vi "Auto_Drive_Test.vi"(8 "Timer?":bool, 9 "Duration":u32=3500, 10 "distance":dbl=88.0 format="%#_13g", 11 "Drive Effort":dbl=1000.0) -> ()   [LabVIEW 2016]
uses:
  <vilib>/Rock Robotics/WPI/SafetyOutput/WPI_SafetyOutputConfigMenu.ctl
panel:
  in  "Max Error":dbl=100.0 format="%#_13g"
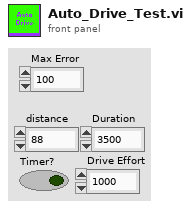
[diagram p1: front panel]
types:
  T1 = typedef "WPI_SafetyOutputConfigMenu.ctl" = enum16{"Enable", "Disable"}
  T2 = typedef "WPI_MotorControlDeviceRef.ctl" = cluster{"DeviceStatus":errorcluster, "Type":T3, "PWM":cluster{"PWM Channel":T4, "DeadBand":T5}, "CAN":cluster{"Device Number":u8, "SetOutput VI Ref":variant, "GetOutput VI Ref":variant, "Enable VI Ref":variant, "Disable VI Ref":variant, "Data":variant}, "Invert":bool}
  T3 = typedef "WPI_MotorControlType.ctl" = enum16{"PWM", "CAN"}
  T4 = typedef "FPGA_DIOPWMChannel.ctl" = enum8{"PWM 0", "PWM 1", "PWM 2", "PWM 3", "PWM 4", "PWM 5", "PWM 6", "PWM 7", "PWM 8", "PWM 9", "PWM MXP 0", "PWM MXP 1", "PWM MXP 2", "PWM MXP 3", "PWM MXP 4", "PWM MXP 5", "PWM MXP 6", "PWM MXP 7", "PWM MXP 8", "PWM MXP 9", "Invalid"}
  T5 = typedef "WPI_PWMDeadband.ctl" = cluster{"Name":string, "maxPositivePwm":i32, "minPositivePwm":i32, "centerPwm":i32, "maxNegativePwm":i32, "minNegativePwm":i32, "angularRange":u16}
  T6 = typedef "WPI_CANTalonSRX_GlobalStatus.ctl" = cluster{"Applied Throttle":dbl, "Module Enabled":bool, "CAN Error":errorcluster, "Closed Loop Error":dbl, "Forward Limit Switch Closed":bool, "Reverse Limit Switch Closed":bool, "Sensor Position":dbl, "Sensor Velocity":dbl, "Current":dbl, "Sticky Fault - Over Temp":bool, "Sticky Fault - Under Voltage":bool, "Sticky Fault - Forward Limit":bool, "Sticky Fault - Reverse Limit":bool, "Sticky Fault - Forward Soft Limit":bool, "Sticky Fault - Reverse Soft Limit":bool, "Brake is Enabled":bool, "Encoder Position":dbl, "Encoder Velocity":dbl, "Encoder Index Count":dbl, "Encoder A Pin State":bool, "Encoder B Pin State":bool, "Encoder Index Pin State":bool, "Analog In":dbl, "Analog In Velocity":dbl, "Temperature (C)":dbl, "Battery Voltage":dbl, "Control 5 Is Supported":bool, "Current Profile Slot Select":dbl, "Pos Div 8":bool, "Vel Div 4":bool, "Pulse Width Position":i32, "Pulse Width Velocity":i32, "Pulse Width Rise To Rise (us)":i32, "Pulse Width Rise To Fall (us)":i32, "Mot Prof Active Is Under Run":bool, "Mot Prof Active Has Under Run":bool, "Mot Prof Active Is Last":bool, "Mot Prof Active Velocity Only":bool, "Mot Prof Active Is Valid":bool, "Mot Prof Buffer Is Full":bool, "Mot Prof Active Profile Slot Select":i32, "Mot Prof NextID":i32, "Mot Prof Count":i32, "Mot Prof Active Velocity":dbl, "Mot Prof Active Position":dbl, "Mot Prof Output Enable":i32}
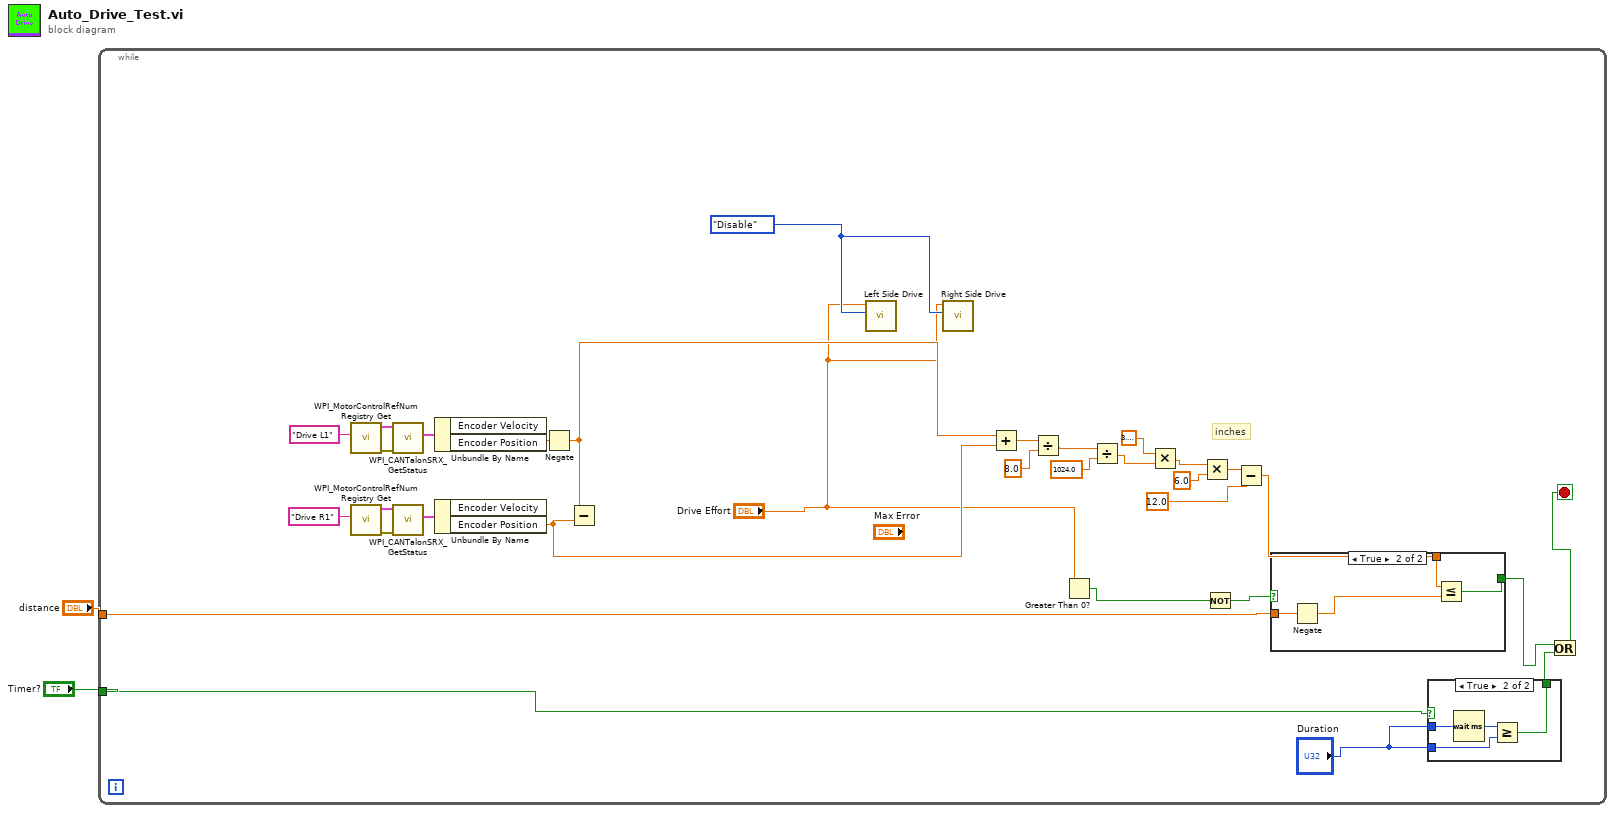
[diagram p0: block diagram]
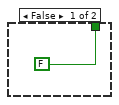
[diagram p2: hidden frame]
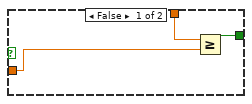
[diagram p3: hidden frame]
diagram:
  n1 = while {
    tunnel: "distance" -> [w18]
    tunnel: "Timer?" -> [w13]
    stop <- w10 stop-if-true
    w4 = WPI_SafetyOutputConfigMenu."Disable" ("mode")
    # "inches"
    n2 = call <vilib>:"WPI_MotorControlRefNum Registry Get.vi"("refnum name"="Drive L1") -> ("error out"=w29:errorcluster, "MotorControlDevRef"=w34:T2)  [unwired: 9 in]
    n3 = call <vilib>:"WPI_MotorControlRefNum Registry Get.vi"("refnum name"="Drive R1") -> ("error out"=w32:errorcluster, "MotorControlDevRef"=w33:T2)  [unwired: 9 in]
    n4 = call <vilib>:"WPI_CANTalonSRX_GetStatus.vi"("error in (no error)"=w29, "CAN Talon SRX Ref"=w34) -> ("Talon SRX Status"=w31:T6)  [unwired: 7 in, 2 out]
    n5 = call <vilib>:"WPI_CANTalonSRX_GetStatus.vi"("error in (no error)"=w32, "CAN Talon SRX Ref"=w33) -> ("Talon SRX Status"=w30:T6)  [unwired: 7 in, 2 out]
    n6 = Unbundle By Name(w31) -> ("Encoder Position"=w6:dbl)  [unwired: 1 out]
    n7 = Unbundle By Name(w30) -> ("Encoder Position"=w7:dbl)  [unwired: 1 out]
    n8 = Negate(x=w6) -> (-x=w5:dbl)
    n9 = Subtract(x=w5, y=w7) -> ()  [unwired: 1 out]
    n10 = call "Left Side Drive.vi"("mode"=w4, "Effort"="Drive Effort") -> ()  [unwired: 10 in]
    n11 = call "Right Side Drive.vi"("mode"=w4, "Effort"="Drive Effort") -> ()  [unwired: 10 in]
    n12 = Add(x=w5, y=w7) -> (x+y=w28:dbl)
    n13 = Divide(x=w28, y=8.0) -> (x/y=w26:dbl)
    n14 = Greater Than 0?(x="Drive Effort") -> (x > 0?=w14:bool)
    n15 = Divide(x=w26, y=1024.0) -> (x/y=w24:dbl)
    n16 = Multiply(x=3.141592653589793, y=w24) -> (x*y=w22:dbl)
    n17 = Multiply(x=w22, y=6.0) -> (x*y=w17:dbl)
    n18 = Not(x=w14) -> (.not. x?=w8:bool)
    n19 = Subtract(x=w17, y=12.0) -> (x-y=w15:dbl)
    n20 = case shown="True" w8 {
      tunnel: [w40 w46] -> w12
      tunnel: w18 -> [w41 w44]
      tunnel: w15 -> [w42 w43]
      frame False {
        n21 = Greater Or Equal?(x=w42, y=w41) -> (x >= y?=w40:bool)
      }
      frame True {
        n22 = Negate(x=w44) -> (-x=w45:dbl)
        n23 = Less Or Equal?(x=w43, y=w45) -> (x <= y?=w46:bool)
      }
    }
    n24 = case shown="True" w13 {
      tunnel: "Duration" -> [_ w38]
      tunnel: [FALSE w37] -> w11
      tunnel: "Duration" -> [_ w36]
      frame False {
      }
      frame True {
        n25 = Wait (ms)(milliseconds to wait=w36) -> (millisecond timer value=w39:u32)
        n26 = Greater Or Equal?(x=w39, y=w38) -> (x >= y?=w37:bool)
      }
    }
    n27 = Or(x=w12, y=w11) -> (x .or. y?=w10:bool)
  }
